vi "NPC3SG Connect v10.6.2.vi"(2 "Calibration File":path, 4 "Drive Port":refnum<visa-resource-name>="COM5" caption="Visa Port") -> (0 "Success":bool, 1 "Drive Visa Name":refnum<visa-resource-name>)   [LabVIEW 2010]
uses:
  drivers/Newport NPC3SG/SubNPC3SG.llb/device variables.vi
panel:
  out "Read Error":errorcluster caption="error out" {"code" format="%x"}
  out "Connection Error":errorcluster
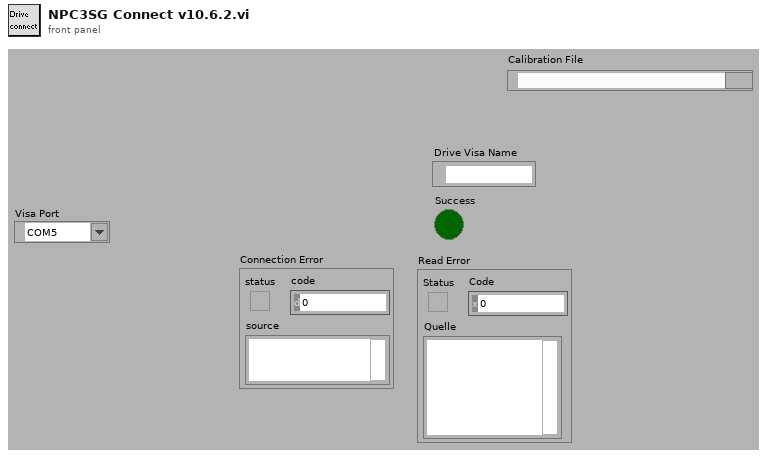
[diagram p1: front panel]
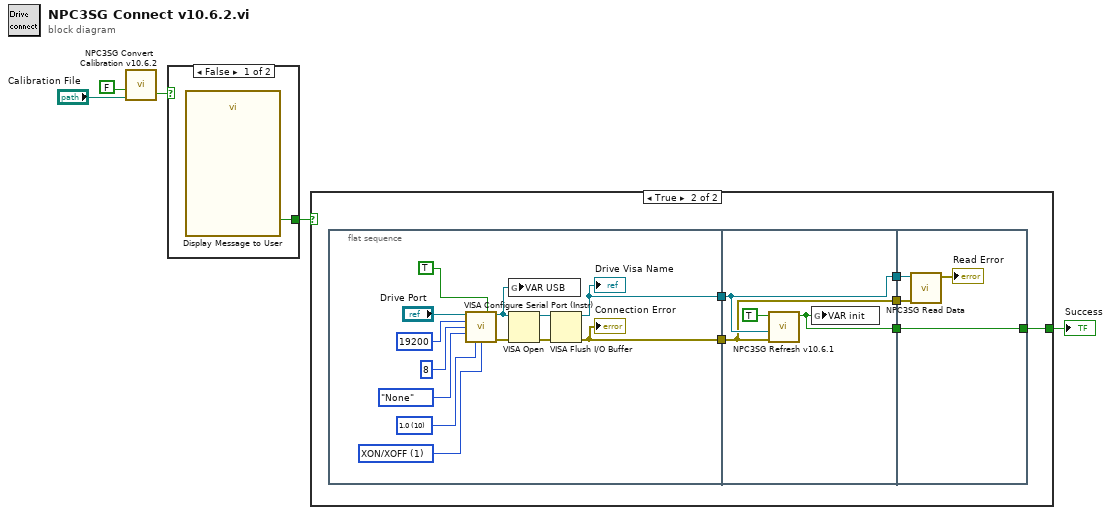
[diagram p0: block diagram]
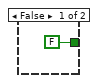
[diagram p2: hidden frame]
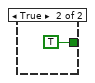
[diagram p3: hidden frame]
diagram:
  n1 = call "NPC3SG Convert Calibration v10.6.2.vi"("Calibration File"="Calibration File", "Is Voltage?"=FALSE) -> ("Has calibration?"=w4:bool)  [unwired: 2 in, 1 out]
  n2 = case shown="False" w4 {
    tunnel: [w6 TRUE ("OK")] -> w2
    frame False {
      n3 = call "Display Message to User"() -> ("OK"=w6:bool)  [unwired: 10 in, 1 out]
    }
    frame True {
    }
  }
  n4 = case shown="True" w2 {
    tunnel: [FALSE ("init ok??") w9] -> w3
    frame False {
    }
    frame True {
      n5 = flat-sequence {
        tunnel: [w17] -> w14
        tunnel: [w16] -> w13
        tunnel: w14 -> [w30]
        tunnel: w13 -> [w29]
        tunnel: [w30] -> w12
        tunnel: [w29] -> w11
        tunnel: [w28] -> w10
        tunnel: w12 -> [w34]
        tunnel: w11 -> [w33]
        tunnel: [w32] -> w9
        tunnel: w10 -> [w32]
        frame #0 {
          w19 = u16 1 items=["Kein", "XON/XOFF", "RTS/CTS", "XON/XOFF & RTS/CTS", "DTR/DSR", "XON/XOFF & DTR/DSR"] ("flow control (0:none)")
          w27 = u16 10 items=["1.0"=10, "1.5"=15, "2.0"=20] ("stop bits (10: 1 bit)")
          n6 = call <vilib>:"VISA Configure Serial Port (Instr).vi"("VISA resource name"="Drive Port", "Enable Termination\nChar (T)"=TRUE ("Enable Termination\nChar (T)"), "baud rate (9600)"=u32 19200, "data bits (8)"=u16 8, "parity (0:none)"=enum16{"None", "Odd", "Even", "Mark", "Space"}."None", "stop bits (10: 1 bit)"=w27, "flow control (0:none)"=w19) -> ("VISA resource name out"=w18:refnum<visa-resource-name>, "error out"=w21:errorcluster)  [unwired: 7 in]
          n7 = global write "device variables.vi" "VAR USB"(w18) -> ()
          n8 = VISA Open(error in (no error)=w21, VISA resource name=w18) -> (VISA resource name=w22:refnum<visa-resource-name>, error out=w23:errorcluster)  [unwired: 3 in]
          n9 = VISA Flush I/O Buffer(VISA resource name=w22, error in (no error)=w23) -> (VISA resource name out=w17:refnum<visa-resource-name>, error out=w16:errorcluster)  [unwired: 1 in]
          "Connection Error" <- w16
          "Drive Visa Name" <- w17
        }
        frame #1 {
          n10 = call "NPC3SG Refresh v10.6.1.vi"("error in"=w29, "VISA-Ressourcen-Name (In)"=w30, "reset all"=TRUE) -> ("init ok??"=w28:bool)  [unwired: 8 in]
          n11 = global write "device variables.vi" "VAR init"(w28) -> ()
        }
        frame #2 {
          n12 = call "NPC3SG Read Data.vi"("VISA resource name in"=w34, "error in"=w33) -> ("error ende"=→"Read Error":errorcluster)  [unwired: 8 in]
        }
      }
    }
  }
  "Success" <- w3
